vi "289_check_config.vi"(8 "error in (no error)":errorcluster, 11 "VISA resource name":refnum<visa-resource-name>) -> (0 "error out":errorcluster, 1 "Range":string, 2 "Escala Principal":string, 3 "VISA resource name out":refnum<visa-resource-name>, 4 "Escala Secundária":string, 5 "Secundária":string)   [LabVIEW 2015, in "289.lvclass"]
uses:
  289.lvclass
panel:
  out "array":string[](array[string])
  out "read buffer":string
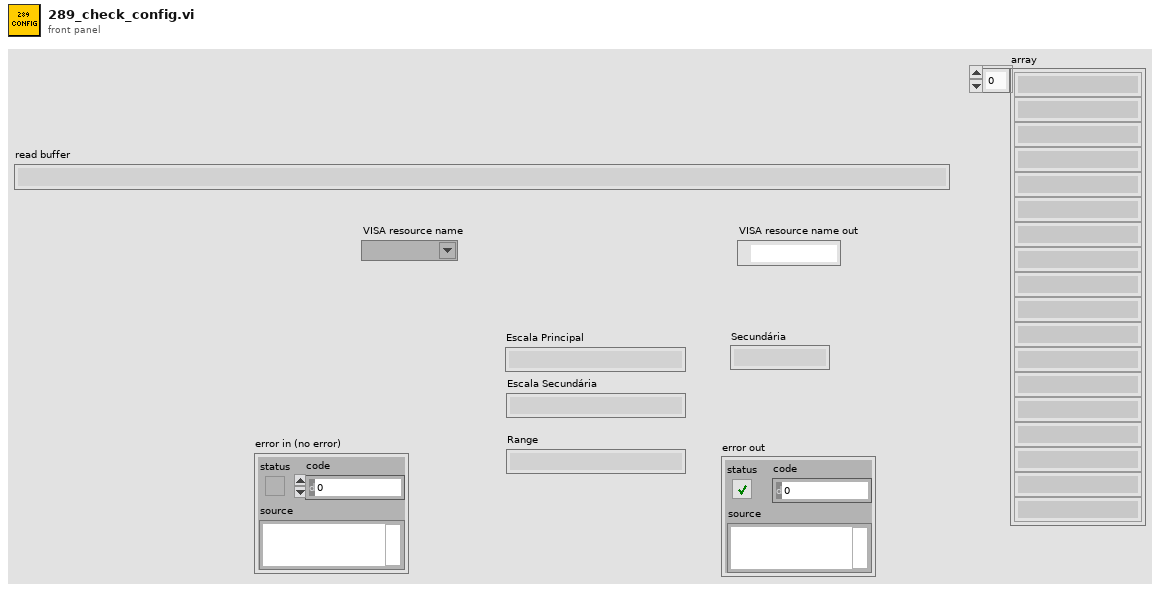
[diagram p1: front panel]
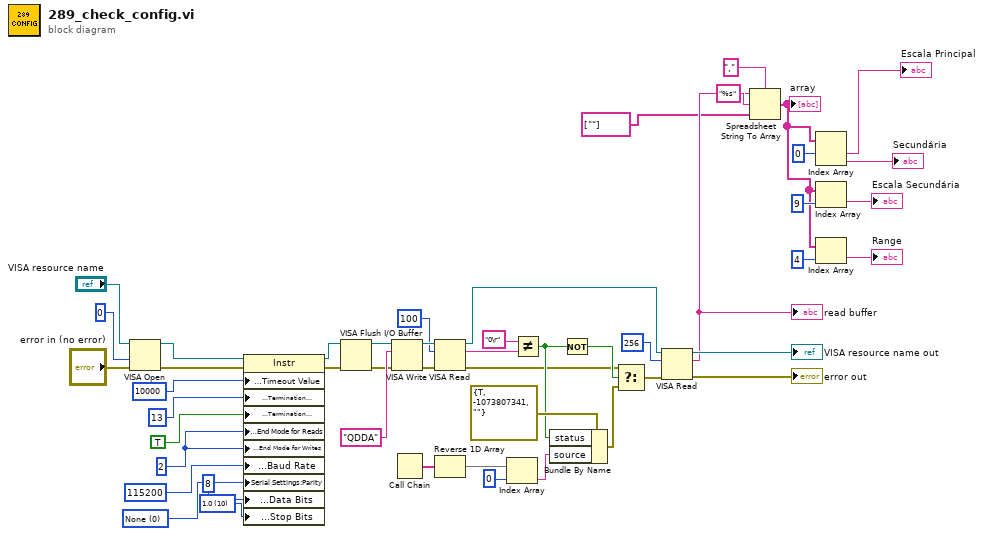
[diagram p0: block diagram]
diagram:
  w38 = u16 10 items=["1.0"=10, "1.5"=15, "2.0"=20] ("Serial Settings:Serial Stop Bits")
  w40 = u16 0 items=["None", "Odd", "Even", "Mark", "Space"] ("Serial Settings:Serial Parity")
  w44 = u16 2 ("ASRL End In")
  n1 = VISA Open(access mode=u32 0, error in (no error)="error in (no error)", VISA resource name="VISA resource name") -> (VISA resource name=w37:refnum<visa-resource-name>, error out=w36:errorcluster)  [unwired: 2 in]
  n2 = property class="Instr"(reference=w37, error in=w36, "General Settings:Timeout Value"=u32 10000, "Message Based Settings:Termination Character"=u8 13 ("TermChar"), "Message Based Settings:Termination Character Enable"=TRUE ("TermChar En"), "Serial Settings:End Mode for Reads"=w44, "Serial Settings:End Mode for Writes"=w44, "Serial Settings:Baud Rate"=u32 115200 ("Serial Settings:Serial Baud Rate"), "Serial Settings:Parity"=w40, "Serial Settings:Data Bits"=u16 8 ("Serial Settings:Serial Data Bits"), "Serial Settings:Stop Bits"=w38) -> (reference out=w43:refnum<visa-resource-name>, error out=w42:errorcluster)
  n3 = VISA Flush I/O Buffer(VISA resource name=w43, error in (no error)=w42) -> (VISA resource name out=w33:refnum<visa-resource-name>, error out=w32:errorcluster)  [unwired: 1 in]
  n4 = VISA Write(VISA resource name=w33, write buffer="QDDA" ("ID Query (QM)"), error in (no error)=w32) -> (VISA resource name out=w20:refnum<visa-resource-name>, error out=w18:errorcluster)  [unwired: 1 out]
  n5 = Call Chain() -> (call chain=w29:string[])
  n6 = VISA Read(VISA resource name=w20, byte count=u32 100 ("Byte Count (0)"), error in (no error)=w18) -> (VISA resource name out=w17:refnum<visa-resource-name>, read buffer=w25:string, error out=w21:errorcluster)  [unwired: 1 out]
  n7 = Reverse 1D Array(array=w29) -> (reversed array=w28:string[])
  n8 = Index Array(array=w28, index=0) -> (element=w27:string)
  n9 = Not Equal?(x="0\r", y=w25) -> (x != y?=w24:bool)
  n10 = Bundle By Name(cluster=errorcluster {"status"=TRUE, "code"=-1073807341, "source"=""} ("t"), "status"=w24, "source"=w27) -> (w22:errorcluster)
  n11 = Not(x=w24) -> (.not. x?=w23:bool)
  n12 = Select(t=w21, s=w23, f=w22) -> (s? t:f=w16:errorcluster)
  n13 = VISA Read(VISA resource name=w17, byte count=u32 256, error in (no error)=w16) -> (VISA resource name out=→"VISA resource name out":refnum<visa-resource-name>, read buffer=w11:string, error out=→"error out":errorcluster)  [unwired: 1 out]
  "read buffer" <- w11
  n14 = Spreadsheet String To Array(delimiter (Tab)="," ("regular expression"), format string="%s", spreadsheet string=w11, array type (2D Dbl)=string[] [""]) -> (array=w2:string[])
  "array" <- w2
  n15 = Index Array(array=w2, index #1=0 ("index")) -> (element #1=→"Escala Principal":string, element #2=→"Secundária":string)  [unwired: 1 in]
  n16 = Index Array(array=w2, index=9) -> (element=→"Escala Secundária":string)
  n17 = Index Array(array=w2, index=4) -> (element=→"Range":string)
